vi "Data.Initialize.vi"(8 "error in (no error)":errorcluster, 11 "Data Access API in":refnum<class "Data Access API.lvclass">) -> (0 "error out":errorcluster, 3 "Data Access API out":refnum<class "Data Access API.lvclass">)   [LabVIEW 2015, in "Data Access API.lvlib" / "Data Access API.lvclass"]
uses:
  Data Access API.lvclass
  Data Access API.lvclass/Data Access API.ctl
  Data/Read/Read.lvclass/Read.ctl
  Data/Read/Read.lvclass
  Data/Write/Write.lvclass/Write.ctl
  Data/Write/Write.lvclass
  Data/ReadWrite/ReadWrite.lvclass/ReadWrite.ctl
  Data/ReadWrite/ReadWrite.lvclass
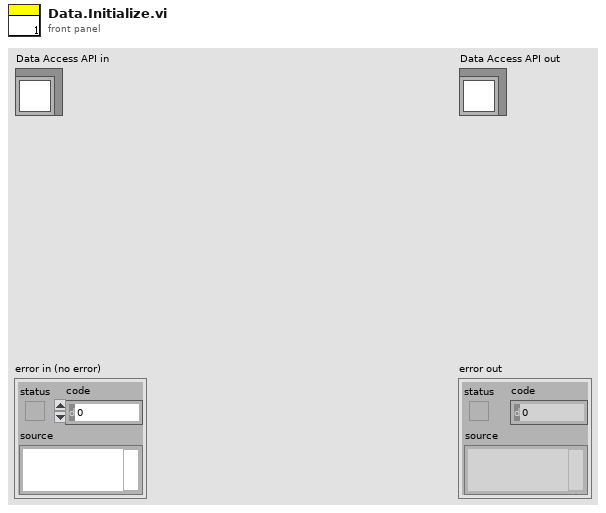
[diagram p1: front panel]
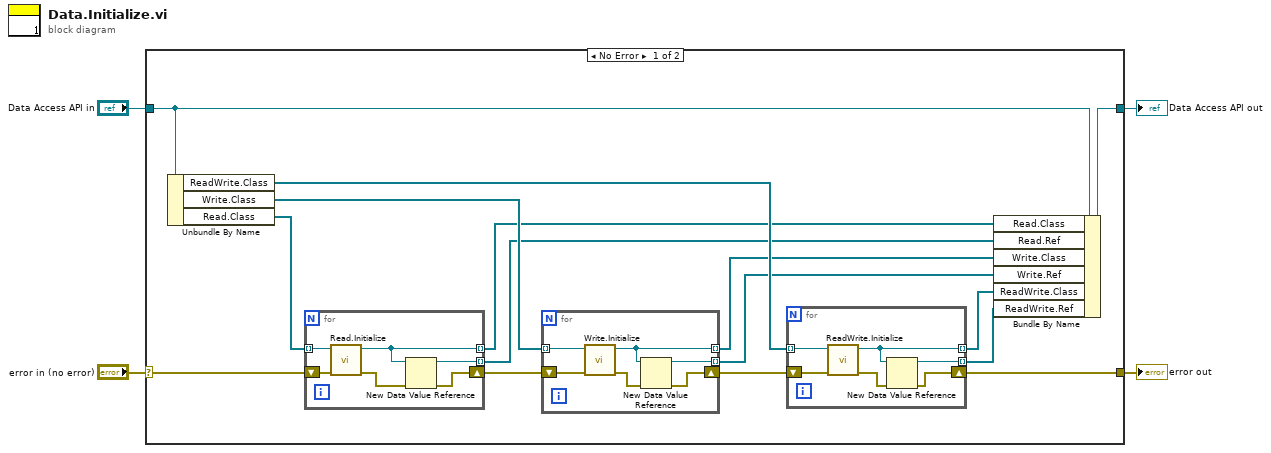
[diagram p0: block diagram]
diagram:
  n1 = case shown="No Error" "error in (no error)" {
    selector: "error in (no error)" -> [w18 w39]
    tunnel: [w15 w39] -> w3
    tunnel: [w8 w38] -> w1
    tunnel: "Data Access API in" -> [w9 w38]
    frame No Error {
      n2 = Unbundle By Name(w9) -> ("ReadWrite.Class"=w13:refnum<class "ReadWrite.lvclass">[], "Write.Class"=w14:refnum<class "Write.lvclass">[], "Read.Class"=w19:refnum<class "Read.lvclass">[])
      n3 = for {
        tunnel: w19 -> [w37] mode=indexing
        shift-right: [w34] -> w17
        shift-left: w18 -> [w36]
        tunnel: [w33] -> w10 mode=indexing
        tunnel: [w32] -> w5 mode=indexing
        n4 = call "Read.Initialize.vi"("error in (no error)"=w36, "Read in"=w37) -> ("error out"=w35:errorcluster, "Read out"=w33:refnum<class "Read.lvclass">)  [unwired: 8 in]
        n5 = New Data Value Reference(data value=w33, error in=w35) -> (data value reference=w32:refnum<data-value>, error out=w34:errorcluster)
      }
      n6 = for {
        tunnel: w14 -> [w31] mode=indexing
        shift-right: [w27] -> w16
        shift-left: w17 -> [w30]
        tunnel: [w29] -> w11 mode=indexing
        tunnel: [w26] -> w6 mode=indexing
        n7 = call "Write.Initialize.vi"("error in (no error)"=w30, "Write in"=w31) -> ("error out"=w28:errorcluster, "Write out"=w29:refnum<class "Write.lvclass">)  [unwired: 8 in]
        n8 = New Data Value Reference(data value=w29, error in=w28) -> (data value reference=w26:refnum<data-value>, error out=w27:errorcluster)
      }
      n9 = for {
        tunnel: w13 -> [w24] mode=indexing
        shift-right: [w22] -> w15
        shift-left: w16 -> [w25]
        tunnel: [w21] -> w12 mode=indexing
        tunnel: [w20] -> w7 mode=indexing
        n10 = call "ReadWrite.Initialize.vi"("error in (no error)"=w25, "ReadWrite in"=w24) -> ("error out"=w23:errorcluster, "ReadWrite out"=w21:refnum<class "ReadWrite.lvclass">)  [unwired: 8 in]
        n11 = New Data Value Reference(data value=w21, error in=w23) -> (data value reference=w20:refnum<data-value>, error out=w22:errorcluster)
      }
      n12 = Bundle By Name(cluster=w9, "Read.Class"=w10, "Read.Ref"=w5, "Write.Class"=w11, "Write.Ref"=w6, "ReadWrite.Class"=w12, "ReadWrite.Ref"=w7) -> (w8:refnum<class "Data Access API.lvclass">)
    }
    frame Error {
    }
  }
  "error out" <- w3
  "Data Access API out" <- w1
